vi "Try Match Response.vi"(8 "error in":errorcluster, 10 "ICAN CC Frame":refnum<class "ICAN CC Frame.lvclass">, 11 "Block Upload Transfer in":refnum<class "Block Upload Sub-Block Transfer.lvclass">) -> (0 "error out":errorcluster, 2 "Match":bool, 3 "SDO Transfer out":refnum<class "SDO Transfer.lvclass">)   [LabVIEW 2020, in "CANopen.lvlib" / "SDO Manager.lvlib" / "Block Upload Sub-Block Transfer.lvclass"]
uses:
  Block Upload Sub-Block Transfer.lvclass
  D:/git/CANopen-LabVIEW/source/SDO Manager/SDO Manager/SDO Transfer/SDO Transfer.lvclass
  D:/git/CANopen-LabVIEW/source/SDO Manager/SDO Manager/Block Upload Initiate Transfer/Block Upload Initiate Transfer.lvclass
  SDO Transfer/SDO Transfer.lvclass
  HAL/Source/Interfaces/ICAN CC Frame/ICAN CC Frame.lvclass
  D:/git/HAL/Source/Interfaces/IMessage/IMessage.lvclass
  SDO Transfer/SDO Transfer.lvclass/SDO Transfer.ctl
  Block Upload Initiate Transfer/Block Upload Initiate Transfer.lvclass/Block Upload Initiate Transfer.ctl
  Block Upload Sub-Block Transfer.lvclass/Block Upload Sub-Block Transfer.ctl
  SDO Manager/Block Upload End Transfer/Block Upload End Transfer.lvclass
  HAL/Source/Interfaces/ICommunicate/ICommunicate.lvclass
  CANopen Message/CANopen Message.lvclass
  SDO Transfer/SDO abort code.ctl
  Block Upload Initiate Transfer/Block Upload Initiate Transfer.lvclass
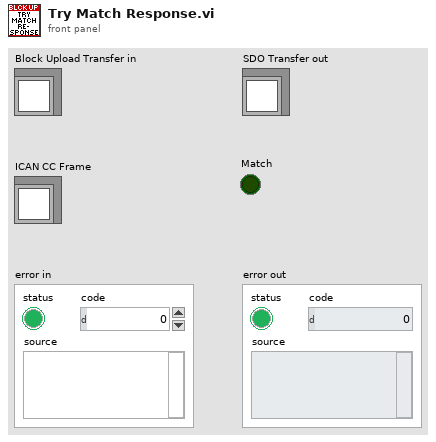
[diagram p1: front panel]
types:
  T1 = typedef "CANopen.lvlib/SDO Manager.lvlib/SDO Transfer.lvclass/SDO abort code.ctl" = u32
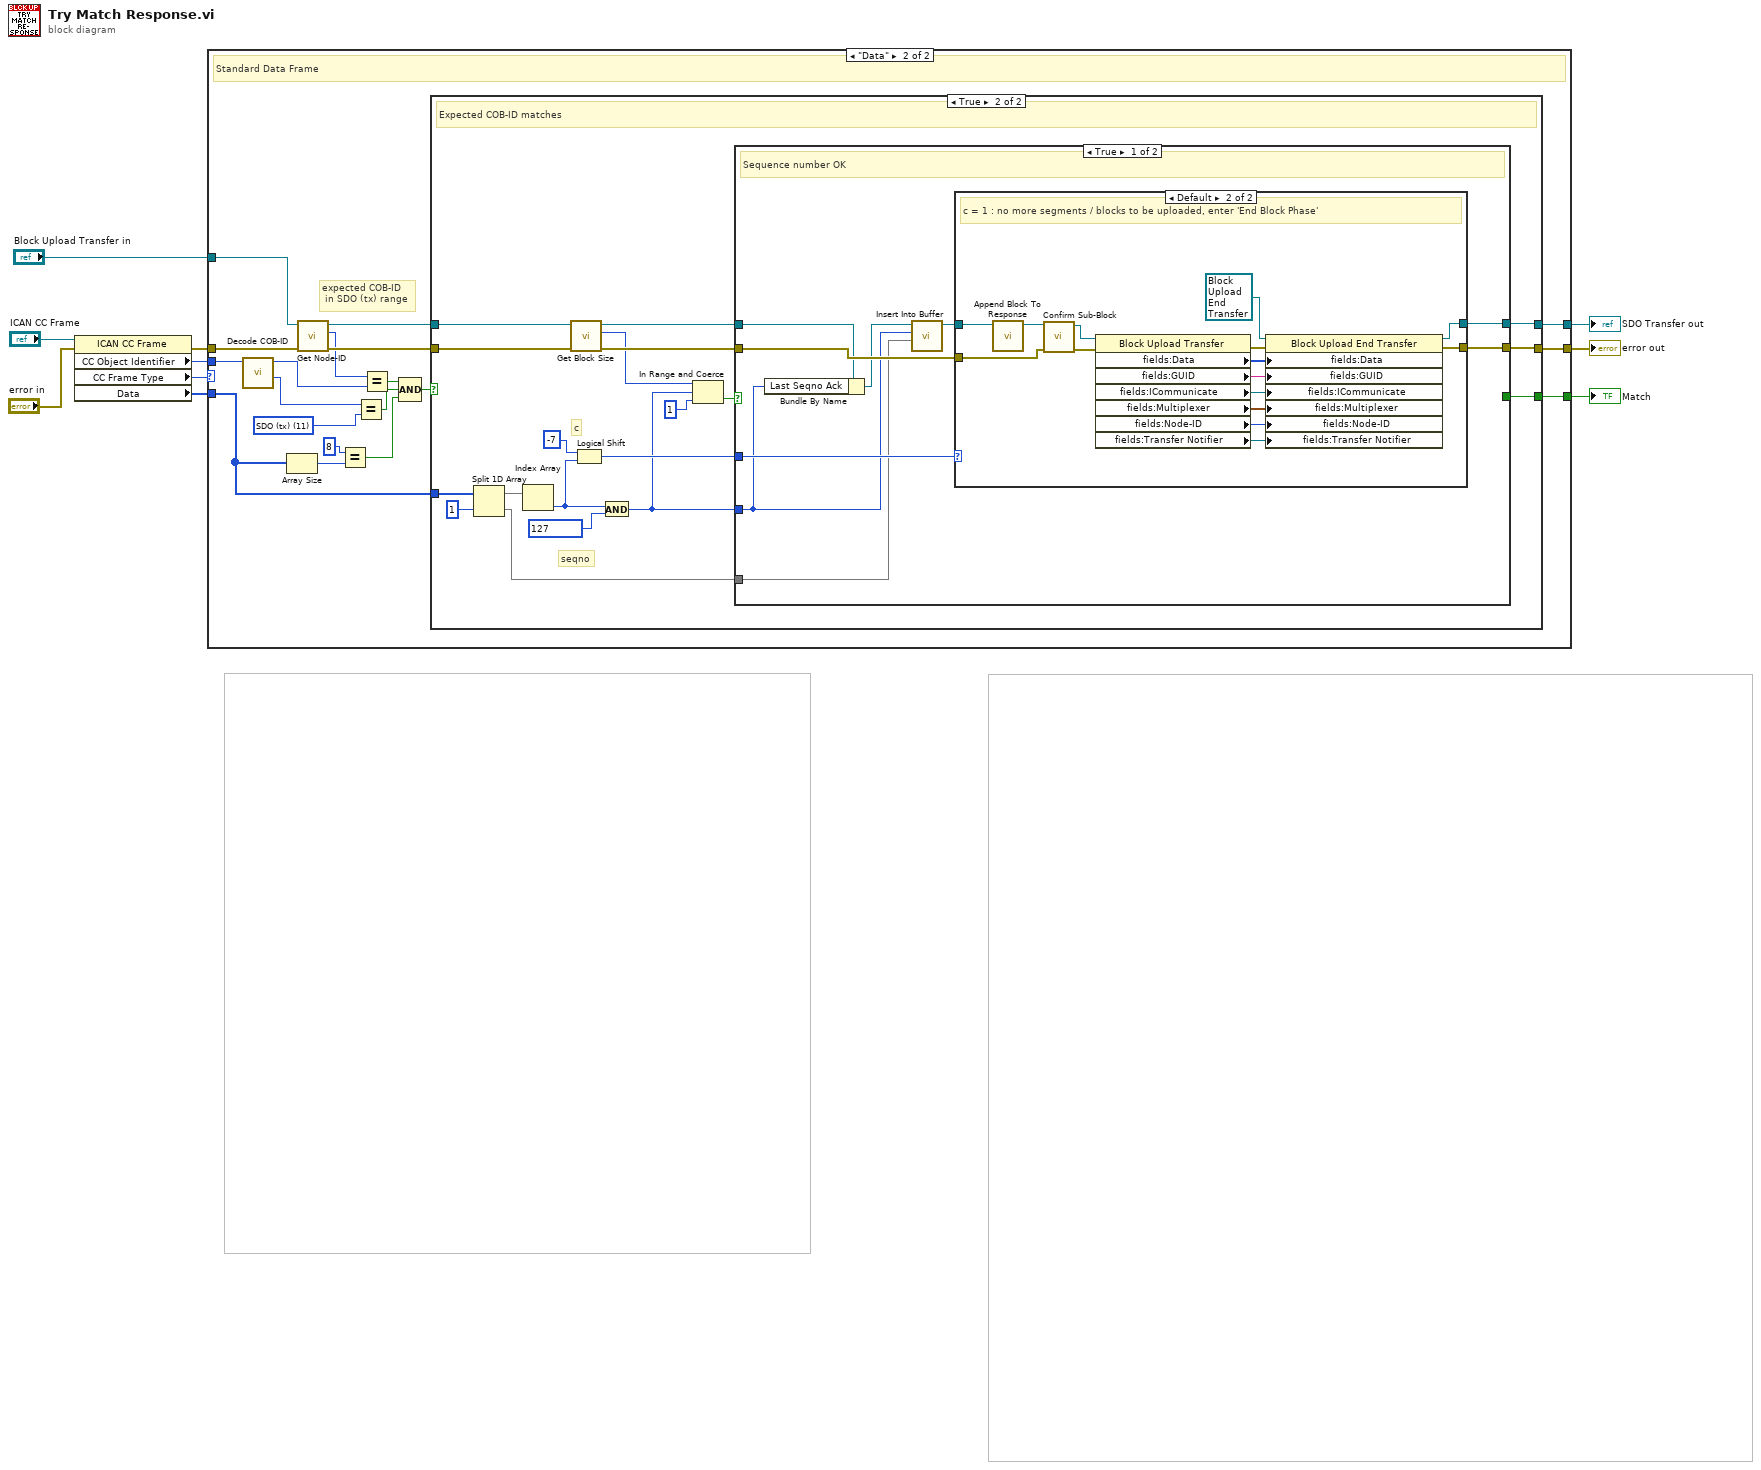
[diagram p0: block diagram]
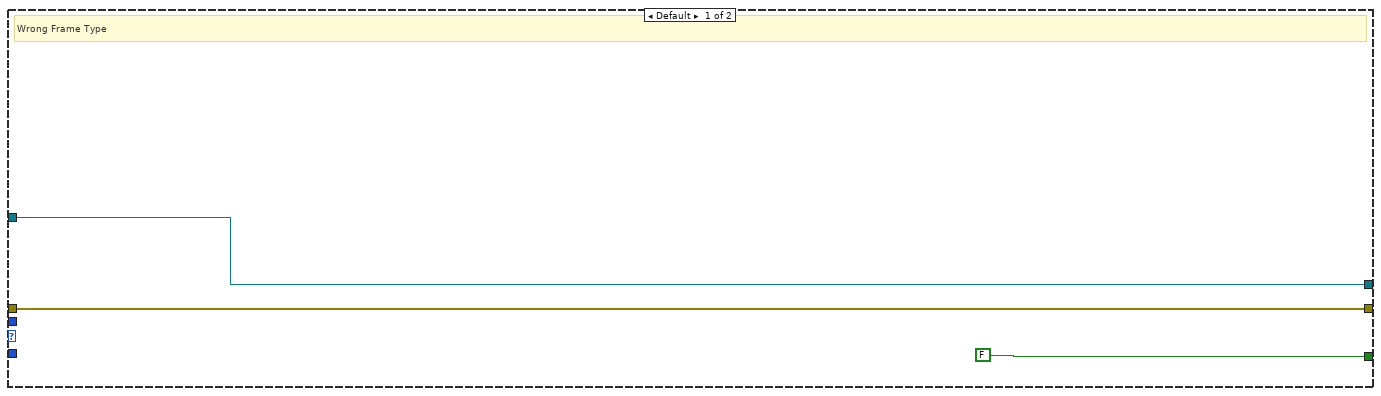
[diagram p2: hidden frame]
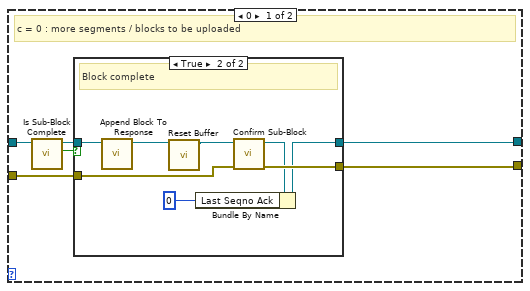
[diagram p4: hidden frame]
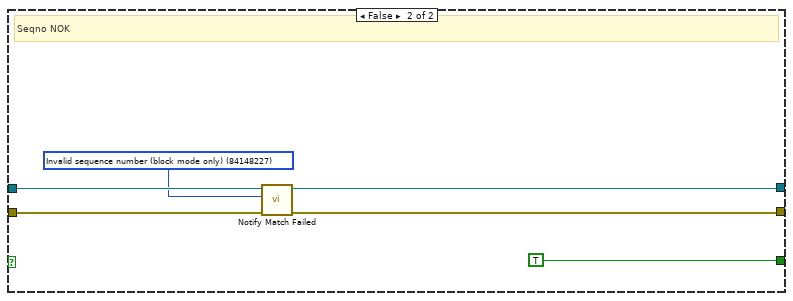
[diagram p6: hidden frame]
diagram:
  n1 = property class="ICAN CC Frame"(reference="ICAN CC Frame", error in="error in") -> (error out=w9:errorcluster, "CC Object Identifier"=w8:u32, "CC Frame Type"=w6:enum8{"Data", "Remote", "Error", "Overload"}, "Data"=w7:u8[])  [unwired: 1 out]
  n2 = case shown="\"Data\"" w6 {
    tunnel: w9 -> [w12 w32]
    tunnel: "Block Upload Transfer in" -> [w11 w31]
    tunnel: [w11 w28] -> w2
    tunnel: [w12 w27] -> w10
    tunnel: [FALSE w26] -> w1
    tunnel: w8 -> [_ w25]
    tunnel: w7 -> [_ w14]
    frame Default {
      # "Wrong Frame Type"
    }
    frame "Data" {
      w22 = u8 11 items=["NMT"=0, "EMCY/SYNC"=1, "TIME"=2, "PDO1 (tx)"=3, "PDO1 (rx)"=4, "PDO2 (tx)"=5, "PDO2 (rx)"=6, "PDO3 (tx)"=7, "PDO3 (rx)"=8, "PDO4 (tx)"=9, "PDO4 (rx)"=10, "SDO (tx)"=11, "SDO (rx)"=12, "NMT error control"=14] ("Function Code")
      # "expected COB-ID\n in SDO (tx) range"
      # "Standard Data Frame"
      n3 = call "Decode COB-ID.vi"("COD-ID"=w25) -> ("Function Code"=w21:u8, "Node-ID"=w24:u8)  [unwired: 9 in]
      n4 = Array Size(array=w14) -> (size(s)=w20:i32)
      n5 = call "Get Node-ID.vi"("error in"=w32, "SDO Transfer in"=w31) -> ("error out"=w29:errorcluster, "Node-ID"=w23:u8, "SDO Transfer out"=w30:refnum<class "Block Upload Sub-Block Transfer.lvclass">)  [unwired: 7 in]
      n6 = Equal?(x=8, y=w20) -> (x = y?=w15:bool)
      n7 = Equal?(x=w21, y=w22) -> (x = y?=w16:bool)
      n8 = Equal?(x=w23, y=w24) -> (x = y?=w17:bool)
      n9 = Compound Arithmetic op=AND(w17, w16, w15) -> (w18:bool)
      n10 = case shown="True" w18 {
        tunnel: w30 -> [w34 w36]
        tunnel: w29 -> [w33 w52]
        tunnel: [w34 w48] -> w28
        tunnel: [w33 w49] -> w27
        tunnel: w14 -> [_ w50]
        tunnel: [_ w47] -> w26
        frame False {
          # "COB-ID mismatch"
        }
        frame True {
          # "seqno"
          # "c"
          # "Expected COB-ID matches"
          n11 = Split 1D Array(array=w50, index=1) -> (first subarray=w44:u8[], second subarray=w45:u8[])
          n12 = Index Array(array=w44) -> (element=w42:u8)  [unwired: 1 in]
          n13 = call "Get Block Size.vi"("error in"=w52, "Block Upload Initiate in"=w36) -> ("error out"=w38:errorcluster, "Block Size"=w37:u8, "Block Upload Initiate out"=w35:refnum<class "Block Upload Sub-Block Transfer.lvclass">)  [unwired: 7 in]
          n14 = Logical Shift(y=i16 -7, x=w42) -> (x << y=w51:u8)
          n15 = And(x=w42, y=u8 127 ("seqno")) -> (x .and. y?=w40:u8)
          n16 = In Range and Coerce(upper limit=w37, x=w40, lower limit=u8 1) -> (In Range?=w39:bool)  [unwired: 1 out]
          n17 = case shown="True" w39 {
            tunnel: w38 -> [w59 w99]
            tunnel: w51 -> [w62 _]
            tunnel: [w61 w98] -> w49
            tunnel: [w60 w96] -> w48
            tunnel: [_ TRUE] -> w47
            tunnel: w45 -> [w57 _]
            tunnel: w35 -> [w56 w97]
            tunnel: w40 -> [w54 _]
            frame True {
              # "Sequence number OK"
              n18 = Bundle By Name(cluster=w56, "Last Seqno Ack"=w54) -> (w55:refnum<class "Block Upload Sub-Block Transfer.lvclass">)
              n19 = call "Insert Into Buffer.vi"("Block"=w57, "Seqno"=w54, "Block Upload Sub-Block Transfer in"=w55) -> ("Block Upload Sub-Block Transfer out"=w58:refnum<class "Block Upload Sub-Block Transfer.lvclass">)  [unwired: 8 in]
              n20 = case shown="Default" w62 {
                tunnel: w58 -> [w65 w81]
                tunnel: w59 -> [w66 w80]
                tunnel: [w67 w85] -> w60
                tunnel: [w68 w92] -> w61
                frame 0 {
                  # "c = 0 : more segments / blocks to be uploaded"
                  n21 = call "Is Sub-Block Complete.vi"("Block Upload Sub-Block Transfer in"=w65) -> ("Complete"=w63:bool, "Block Upload Sub-Block Transfer out"=w64:refnum<class "Block Upload Sub-Block Transfer.lvclass">)  [unwired: 9 in]
                  n22 = case shown="True" w63 {
                    tunnel: w66 -> [w69 w78]
                    tunnel: [w69 w77] -> w68
                    tunnel: [w70 w72] -> w67
                    tunnel: w64 -> [w70 w75]
                    frame False {
                      # "Block incomplete"
                    }
                    frame True {
                      # "Block complete"
                      n23 = call "Append Block To Response.vi"("Block Upload Sub-Block Transfer in"=w75) -> ("Block Upload Sub-Block Transfer out"=w74:refnum<class "Block Upload Sub-Block Transfer.lvclass">)  [unwired: 10 in]
                      n24 = call "Reset Buffer.vi"("Block Upload Sub-Block Transfer in"=w74) -> ("Block Upload Sub-Block Transfer out"=w73:refnum<class "Block Upload Sub-Block Transfer.lvclass">)  [unwired: 10 in]
                      n25 = call "Confirm Sub-Block.vi"("error in"=w78, "Block Upload Sub-Block Transfer in"=w73) -> ("error out"=w77:errorcluster, "Block Upload Sub-Block Transfer out"=w76:refnum<class "Block Upload Sub-Block Transfer.lvclass">)  [unwired: 8 in]
                      n26 = Bundle By Name(cluster=w76, "Last Seqno Ack"=u8 0) -> (w72:refnum<class "Block Upload Sub-Block Transfer.lvclass">)
                    }
                  }
                }
                frame Default {
                  # "c = 1 : no more segments / blocks to be uploaded, enter 'End Block Phase'"
                  n27 = call "Append Block To Response.vi"("Block Upload Sub-Block Transfer in"=w81) -> ("Block Upload Sub-Block Transfer out"=w79:refnum<class "Block Upload Sub-Block Transfer.lvclass">)  [unwired: 10 in]
                  n28 = call "Confirm Sub-Block.vi"("error in"=w80, "Block Upload Sub-Block Transfer in"=w79) -> ("error out"=w84:errorcluster, "Block Upload Sub-Block Transfer out"=w83:refnum<class "Block Upload Sub-Block Transfer.lvclass">)  [unwired: 8 in]
                  n29 = property class="Block Upload Transfer"(reference=w83, error in=w84) -> (error out=w91:errorcluster, "fields:Data"=w82:u8[], "fields:GUID"=w90:string, "fields:ICommunicate"=w89:refnum<class "ICommunicate.lvclass">, "fields:Multiplexer"=w88:cluster{"Index":u16, "Sub-Index":u8}, "fields:Node-ID"=w87:u8, "fields:Transfer Notifier"=w86:refnum<notifier>)  [unwired: 1 out]
                  n30 = property class="Block Upload End Transfer"(reference=refnum<class "Block Upload End Transfer.lvclass"> refnum ("CANopen.lvlib:SDO Manager.lvlib:Block Upload End Transfer"), error in=w91, "fields:Data"=w82, "fields:GUID"=w90, "fields:ICommunicate"=w89, "fields:Multiplexer"=w88, "fields:Node-ID"=w87, "fields:Transfer Notifier"=w86) -> (reference out=w85:refnum<class "Block Upload End Transfer.lvclass">, error out=w92:errorcluster)
                }
              }
            }
            frame False {
              w95 = T1 84148227 items=["Toggle bit not allowed"=84082688, "SDO protocol timed out"=84148224, "Client/server command specifier not valid or unknown"=84148225, "Invalid block size (block mode only)"=84148226, "Invalid sequence number (block mode only)"=84148227, "CRC error (block mode only)"=84148228, "Out of memory"=84148229, "Attempt to read a write only object"=100728833, "Attempt to write a read only object"=100728834, "Object does not exist in the object dictionary"=100794368, "Object cannot be mapped to the PDO"=100925505, "The number and length of the objects to be mapped would exceed PDO length"=100925506, "General parameter incompatibility reason"=100925507, "General internal incompatibility in the device"=100925511, "Access failed due to an hardware error"=101056512, "Data type does not match, length of service parameter does not match"=101122064, "Data type does not match, length of service parameter too high"=101122066, "Data type does not match, length of service parameter too low"=101122067, "Sub-index does not exist"=101253137, "Invalid value for parameter (download only)"=101253168, "Value of parameter written too high (download only)"=101253169, "Value of parameter written too low (download only)"=101253170, "Maximum value is less than minimum value"=101253174, "Resource not available: SDO connection"=101318691, "General error"=134217728, "Data cannot be transferred or stored to the application"=134217760, "Data cannot be transferred or stored to the application because of local control"=134217761, "Data cannot be transferred or stored to the application because of the present device stable"=134217762, "Object dictionary dynamic generation fails or no object dictionary is present (e.g. object dictionary is generated from file and generation fails because of an file error)"=134217763, "No data available"=134217764] ("SDO abort code")
              # "Seqno NOK"
              n31 = call "Notify Match Failed.vi"("error in"=w99, "SDO abort code"=w95, "SDO Transfer in"=w97) -> ("error out"=w98:errorcluster, "SDO Transfer out"=w96:refnum<class "Block Upload Sub-Block Transfer.lvclass">)  [unwired: 7 in]
            }
          }
        }
      }
    }
  }
  "SDO Transfer out" <- w2
  "error out" <- w10
  "Match" <- w1
